vi "get cursor window subarray.vi"(9 "whatever":dbl[](array[numeric]), 10 "omega":dbl[](array[numeric]), 11 "Cursor List":T1) -> (1 "whatever out":dbl[](array[numeric]), 2 "omega out":dbl[](array[numeric]))   [LabVIEW 2010]
uses:
  <vilib>/Utility/miscctls.llb/LVCursorListTypeDef.ctl
panel:
  out "window":dbl=43.07095343680703
  out "left":dbl=2378.60310421286
  out "right":dbl=2421.6740576496672
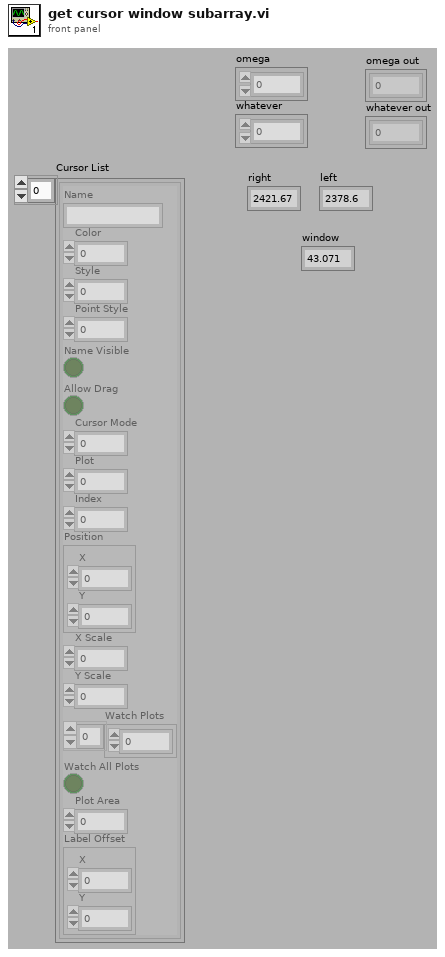
[diagram p1: front panel]
types:
  T1 = typedef "LVCursorListTypeDef.ctl" = cluster{"Name":string, "Color":u32, "Style":u8, "Point Style":u8, "Name Visible":bool, "Allow Drag":bool, "Cursor Mode":u32, "Plot":i32, "Index":i32, "Position":cluster{"X":dbl, "Y":dbl}, "X Scale":u32, "Y Scale":u32, "Watch Plots":i32[], "Watch All Plots":bool, "Plot Area":i32, "Label Offset":cluster{"X":dbl, "Y":dbl}}[]
  T2 = cluster{"Name":string, "Color":u32, "Style":u8, "Point Style":u8, "Name Visible":bool, "Allow Drag":bool, "Cursor Mode":u32, "Plot":i32, "Index":i32, "Position":cluster{"X":dbl, "Y":dbl}, "X Scale":u32, "Y Scale":u32, "Watch Plots":i32[], "Watch All Plots":bool, "Plot Area":i32, "Label Offset":cluster{"X":dbl, "Y":dbl}}
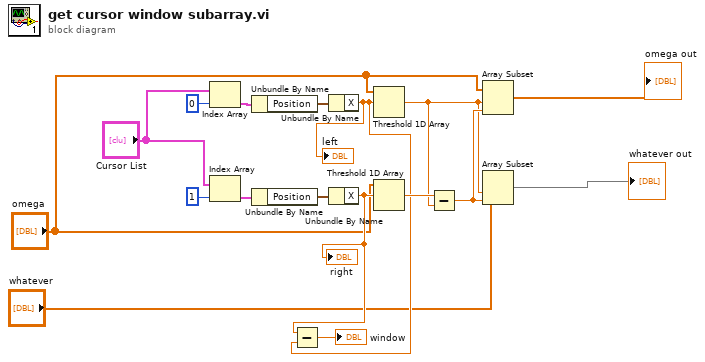
[diagram p0: block diagram]
diagram:
  n1 = Index Array(array="Cursor List", index=0 ("disabled index (col)")) -> (element=w15:T2)
  n2 = Index Array(array="Cursor List", index=1 ("disabled index (col)")) -> (element=w12:T2)
  n3 = Unbundle By Name(w15) -> ("Position"=w14:cluster{"X":dbl, "Y":dbl})
  n4 = Unbundle By Name(w12) -> ("Position"=w11:cluster{"X":dbl, "Y":dbl})
  n5 = Unbundle By Name(w14) -> ("X"=w9:dbl)
  "left" <- w9
  n6 = Unbundle By Name(w11) -> ("X"=w10:dbl)
  "right" <- w10
  n7 = Subtract(x=w10, y=w9) -> (x-y=→"window":dbl)
  n8 = Threshold 1D Array(2:w9, 3:"omega") -> (0:w6:dbl)  [unwired: 1 in]
  n9 = Threshold 1D Array(2:w10, 3:"omega") -> (0:w17:dbl)  [unwired: 1 in]
  n10 = Subtract(x=w17, y=w6) -> (x-y=w7:dbl)
  n11 = Array Subset(array="omega", index=w6, length=w7) -> (→"omega out":dbl[])
  n12 = Array Subset(array="whatever", index=w6, length=w7) -> (→"whatever out":dbl[])
